vi "Poll for Live View Frame.vi"(8 "error in (no error)":errorcluster, 9 "Imaq Image pointer":T1, 10 "Camera State In":T2 {"Sub Region"."V Size"."Value" min=0 max=0 step=4; "Sub Region"."H Size"."Value" min=0 max=0 step=4; "Sub Region"."V Offset"."Value" min=0 max=0 step=4; "Sub Region"."H Offset"."Value" min=0 max=0 step=4}, 11 "Image Data Notifier":refnum<notifier>) -> (0 "error in (no error) 2":errorcluster, 2 "Camera State Out":T2 {"Sub Region"."V Size"."Value" min=0 max=0 step=4; "Sub Region"."H Size"."Value" min=0 max=0 step=4; "Sub Region"."V Offset"."Value" min=0 max=0 step=4; "Sub Region"."H Offset"."Value" min=0 max=0 step=4}, 3 "New Frame?":bool)   [LabVIEW 2015, in "Camera.lvlib"]
uses:
  Camera.lvlib
  Camera State.ctl
  Camera Loop State.ctl
  <vilib>/Utility/miscctls.llb/LVMinMaxIncTypeDef.ctl
  Acquisition Settings.ctl
  Live View State.ctl
  <vilib>/vision/Image Controls.llb/IMAQ Image.ctl
panel:
  out "Frames Per Second":dbl
  out "Image":u16[][](graph)
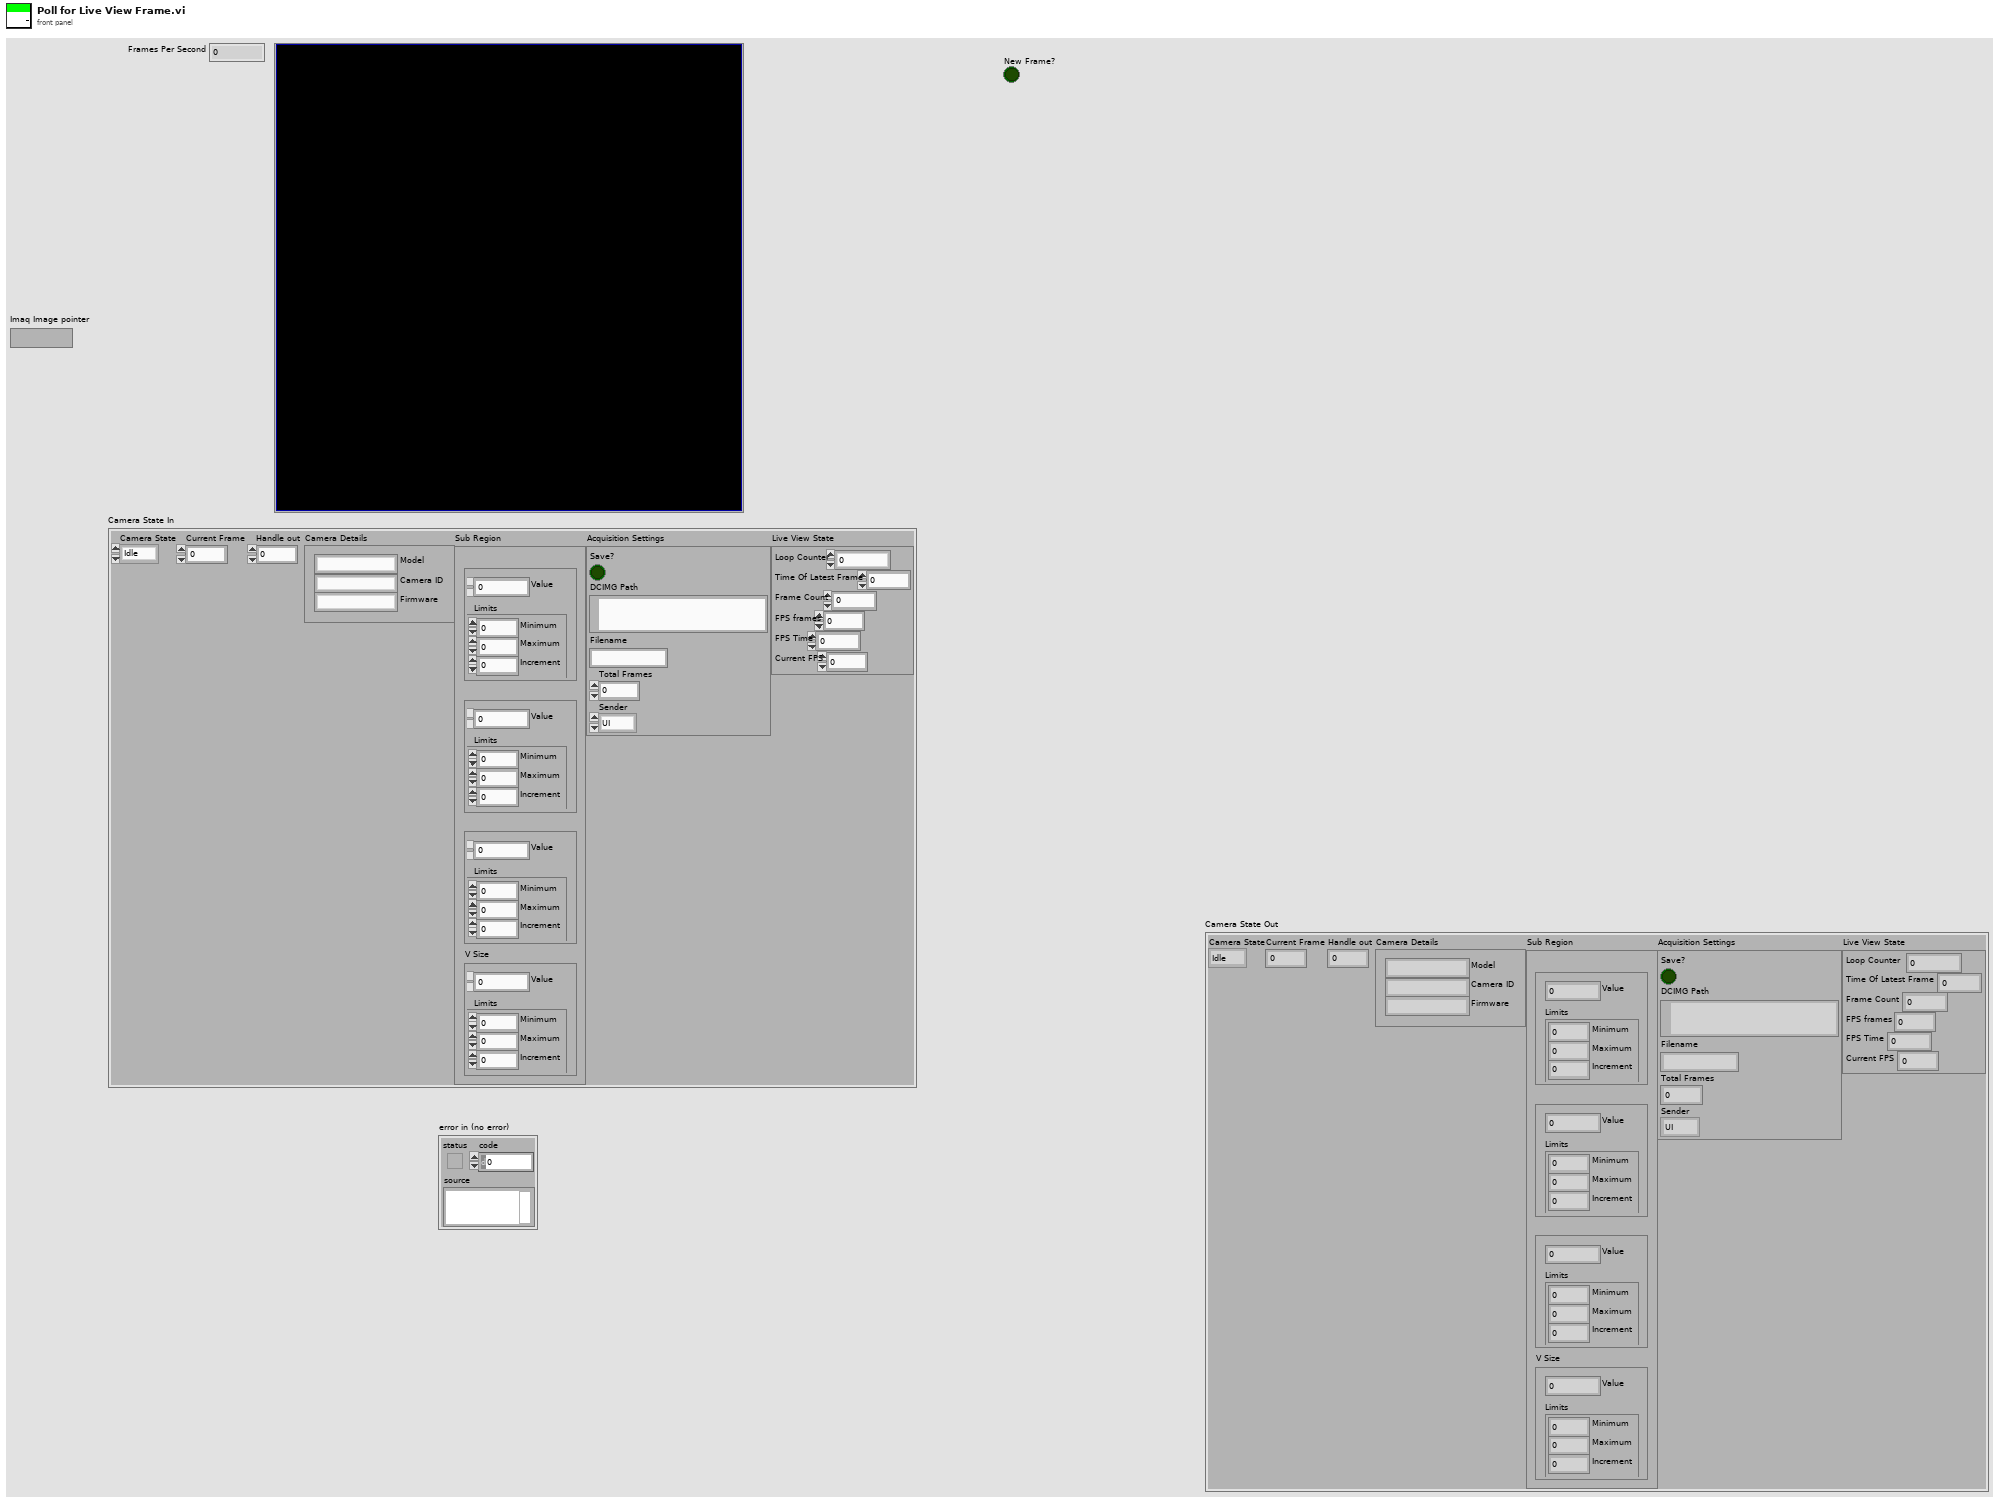
[diagram p1: front panel]
types:
  T1 = typedef "IMAQ Image.ctl" = refnum<image>
  T2 = typedef "Camera.lvlib/Camera State.ctl" = cluster{"Camera State":T3, "Current Frame":i32, "Handle out":u32, "Camera Details":cluster{"Model":string, "Camera ID":string, "Firmware":string}, "Sub Region":cluster{"H Offset":cluster{"Value":i32, "Limits":T4}, "V Offset":cluster{"Value":i32, "Limits":T4}, "H Size":cluster{"Value":i32, "Limits":T4}, "V Size":cluster{"Value":i32, "Limits":T4}}, "Acquisition Settings":T5, "Live View State":T6}
  T3 = typedef "Camera.lvlib/Camera Loop State.ctl" = enum16{"Idle", "Live View", "Ready", "Acquiring"}
  T4 = typedef "LVMinMaxIncTypeDef.ctl" = cluster{"Minimum":dbl, "Maximum":dbl, "Increment":dbl}
  T5 = typedef "Camera.lvlib/Acquisition Settings.ctl" = cluster{"Save?":bool, "DCIMG Path":path, "Filename":string, "Total Frames":i32, "Sender":enum16{"UI", "Automation"}}
  T6 = typedef "Camera.lvlib/Live View State.ctl" = cluster{"Loop Counter":i32, "Time Of Latest Frame":u32, "Frame Count":u32, "FPS frames":dbl, "FPS Time":u32, "Current FPS":dbl}
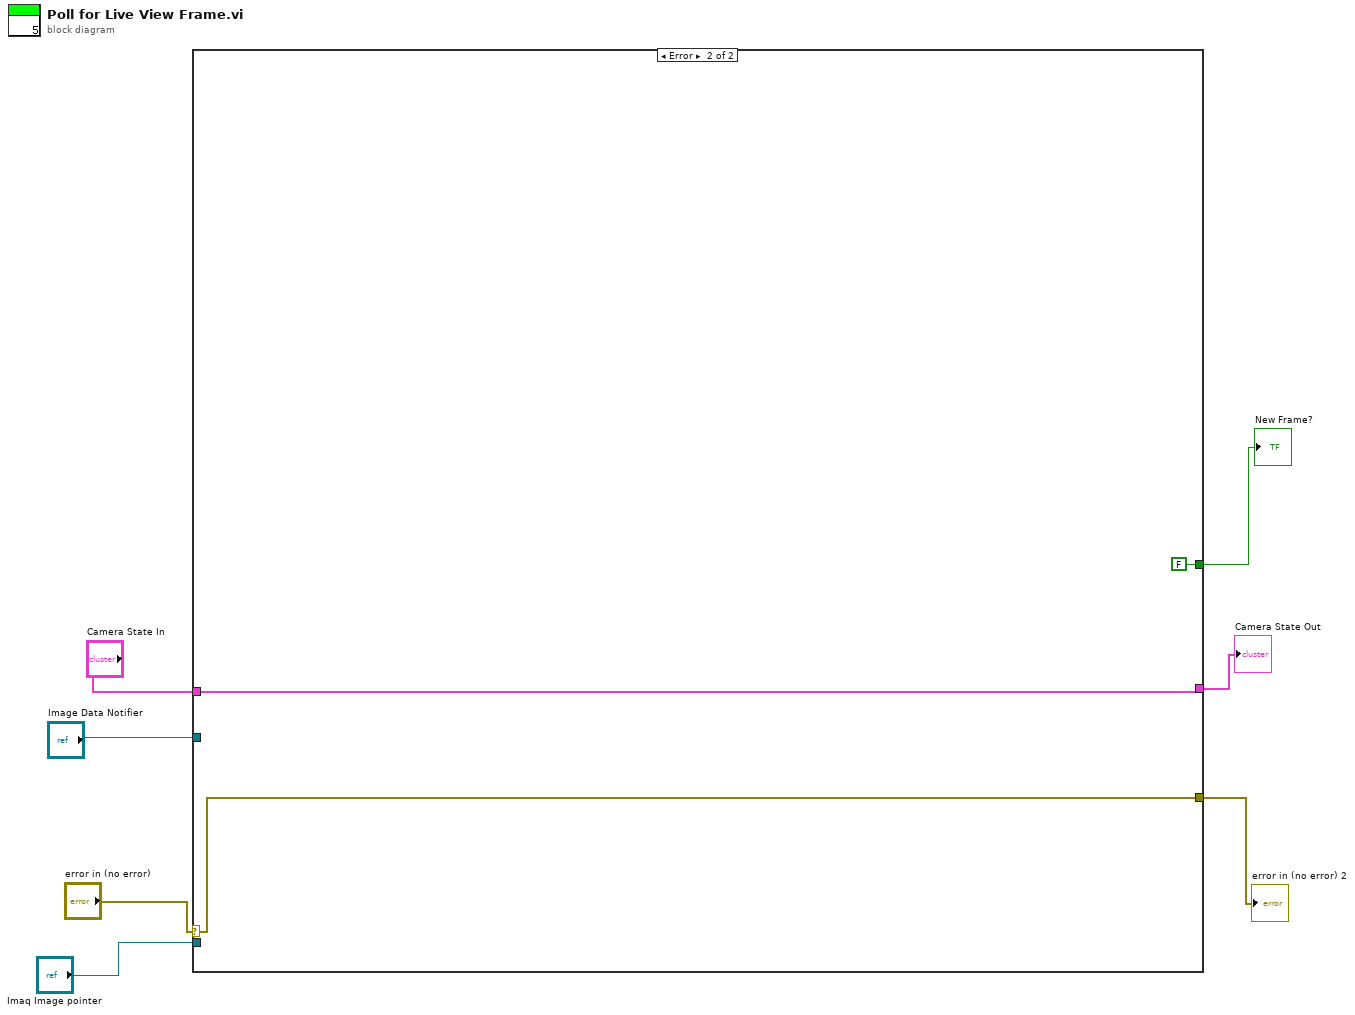
[diagram p0: block diagram]
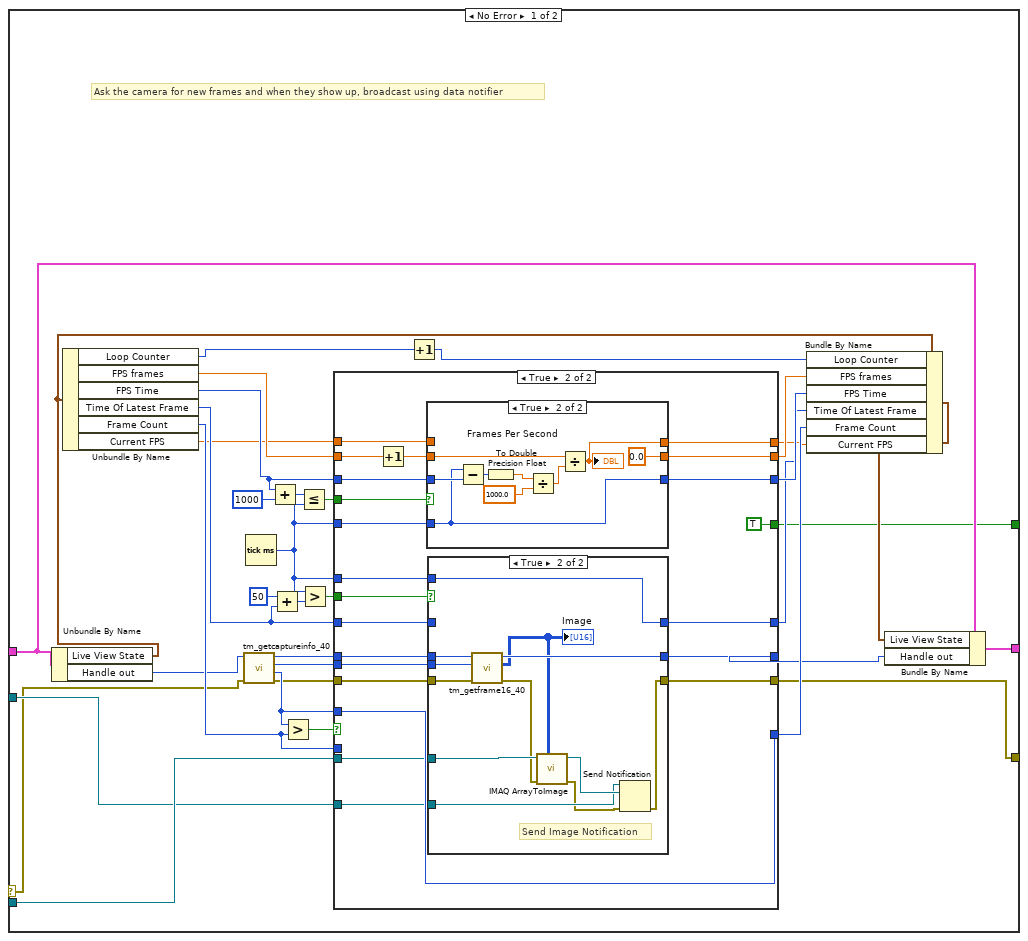
[diagram p2: hidden frame]
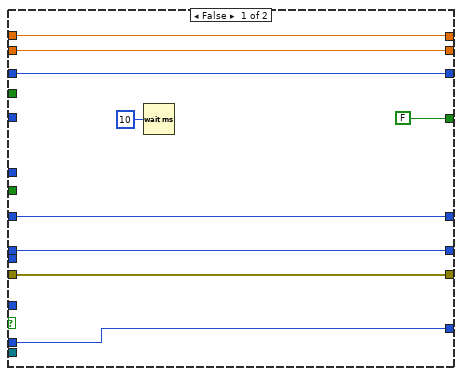
[diagram p3: hidden frame]
diagram:
  n1 = case shown="Error" "error in (no error)" {
    selector: "error in (no error)" -> [w9 w103]
    tunnel: "Camera State In" -> [w15 w102]
    tunnel: "Image Data Notifier" -> [w13 _]
    tunnel: [w20 w103] -> w4
    tunnel: "Imaq Image pointer" -> [w14 _]
    tunnel: [w16 w102] -> w2
    tunnel: [w8 FALSE ("New Frame?")] -> w1
    frame No Error {
      # "Ask the camera for new frames and when they show up, broadcast using data notifier"
      n2 = Unbundle By Name(w15) -> ("Live View State"=w17:T6, "Handle out"=w12:u32)
      n3 = Unbundle By Name(w17) -> ("Loop Counter"=w30:i32, "FPS frames"=w23:dbl, "FPS Time"=w22:u32, "Time Of Latest Frame"=w21:u32, "Frame Count"=w24:u32, "Current FPS"=w10:dbl)
      n4 = call <userlib>:"tm_getcaptureinfo_40.vi"("error in (no error)"=w9, "Handle in"=w12) -> ("error out"=w39:errorcluster, "Frame Count"=w41:i32, "Frame Index"=w38:i32, "Handle out"=w40:u32)  [unwired: 6 in]
      n5 = Tick Count (ms)() -> (millisecond timer value=w33:u32)
      n6 = Add(x=w22, y=u32 1000) -> (x+y=w34:u32)
      n7 = Add(x=u32 50, y=w21) -> (x+y=w37:u32)
      n8 = Greater?(x=w41, y=w24) -> (0:w42:bool)
      n9 = Less Or Equal?(x=w34, y=w33) -> (x <= y?=w31:bool)
      n10 = Greater?(x=w33, y=w37) -> (0:w32:bool)
      n11 = case shown="True" w42 {
        tunnel: w24 -> [w51 _]
        tunnel: [w51 w59] -> w25
        tunnel: w41 -> [_ w59]
        tunnel: w40 -> [w49 w73]
        tunnel: w39 -> [w50 w71]
        tunnel: w38 -> [_ w72]
        tunnel: [w50 w67] -> w20
        tunnel: [w49 w68] -> w19
        tunnel: w22 -> [w47 w70]
        tunnel: w21 -> [w48 w69]
        tunnel: [w48 w66] -> w26
        tunnel: [w47 w65] -> w27
        tunnel: w23 -> [w46 w57]
        tunnel: [w46 w64] -> w28
        tunnel: w33 -> [_ w63]
        tunnel: w33 -> [_ w62]
        tunnel: w32 -> [_ w61]
        tunnel: w31 -> [_ w60]
        tunnel: w14 -> [_ w56]
        tunnel: w13 -> [_ w55]
        tunnel: [w44 w54] -> w11
        tunnel: w10 -> [w44 w53]
        tunnel: [FALSE ("New Frame?") TRUE ("New Frame?")] -> w8
        frame False {
          n12 = Wait (ms)(milliseconds to wait=u32 10) -> ()  [unwired: 1 out]
        }
        frame True {
          n13 = Increment(x=w57) -> (x+1=w58:dbl)
          n14 = case shown="True" w60 {
            tunnel: w70 -> [w91 w95]
            tunnel: [w91 w93] -> w65
            tunnel: w58 -> [w90 w98]
            tunnel: w63 -> [_ w93]
            tunnel: [w90 0.0] -> w64
            tunnel: [w89 w92] -> w54
            tunnel: w53 -> [w89 _]
            frame False {
            }
            frame True {
              n15 = Subtract(x=w93, y=w95) -> (x-y=w94:u32)
              n16 = To Double Precision Float(number=w94) -> (double precision float=w100:dbl)
              n17 = Divide(x=w100, y=1000.0) -> (x/y=w97:dbl)
              n18 = Divide(x=w98, y=w97) -> (x/y=w92:dbl)
              "Frames Per Second" <- w92
            }
          }
          n19 = case shown="True" w61 {
            tunnel: w73 -> [w76 w88]
            tunnel: w71 -> [w75 w87]
            tunnel: w72 -> [_ w86]
            tunnel: w69 -> [w74 _]
            tunnel: w62 -> [_ w85]
            tunnel: [w76 w84] -> w68
            tunnel: [w75 w77] -> w67
            tunnel: [w74 w85] -> w66
            tunnel: w56 -> [_ w82]
            tunnel: w55 -> [_ w79]
            frame False {
            }
            frame True {
              # "Send Image Notification"
              n20 = call <userlib>:"tm_getframe16_40.vi"("error in (no error)"=w87, "Frame Index"=w86, "Handle in"=w88) -> ("error out"=w81:errorcluster, "Data"=w83:u16[][], "Handle out"=w84:u32)  [unwired: 5 in, 1 out]
              "Image" <- w83
              n21 = call "IMAQ ArrayToImage"("Image Pixels (U16)"=w83, "error in (no error)"=w81, "Image"=w82) -> ("error out"=w78:errorcluster, "Image Out"=w80:T1)  [unwired: 7 in]
              n22 = Send Notification(notification=w80, notifier=w79, error in (no error)=w78) -> (error out=w77:errorcluster)  [unwired: 1 out]
            }
          }
        }
      }
      n23 = Increment(x=w30) -> (x+1=w29:i32)
      n24 = Bundle By Name(cluster=w17, "Loop Counter"=w29, "FPS frames"=w28, "FPS Time"=w27, "Time Of Latest Frame"=w26, "Frame Count"=w25, "Current FPS"=w11) -> (w18:T6)
      n25 = Bundle By Name(cluster=w15, "Live View State"=w18, "Handle out"=w19) -> (w16:T2)
    }
    frame Error {
    }
  }
  "error in (no error) 2" <- w4
  "Camera State Out" <- w2
  "New Frame?" <- w1
